vi "HTML Report Text Tag Attribute.vi"(0 "filter value (T)":bool=TRUE, 4 "default value (\"\")":string, 5 "value":string, 6 "label":string, 7 "tag attributes in":string) -> (3 "tag attributes out":string)   [LabVIEW 2020, in "NI_ReportGenerationCore.lvlib"]
doc: "For a value not equal to the default value, constructs the appropriate attribute."
uses:
  <vilib>/Utility/NIReport.llb/NI_ReportGenerationCore.lvlib
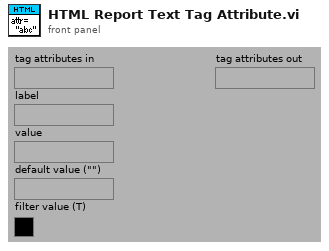
[diagram p1: front panel]
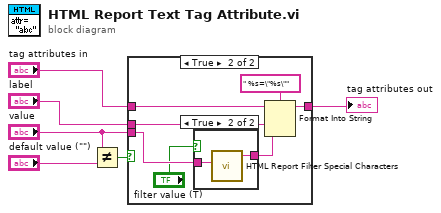
[diagram p0: block diagram]
diagram:
  n1 = Not Equal?(x="value", y="default value (\"\")") -> (x != y?=w3:bool)
  n2 = case shown="True" w3 {
    tunnel: [w7 w14] -> w5
    tunnel: "tag attributes in" -> [w7 w13]
    tunnel: "value" -> [_ w9]
    tunnel: "label" -> [_ w11]
    frame False {
    }
    frame True {
      n3 = case shown="True" "filter value (T)" {
        tunnel: w9 -> [w15 w17]
        tunnel: [w15 w16] -> w10
        frame False {
        }
        frame True {
          n4 = call <vilib>:"HTML Report Filter Special Characters.vi"("character string"=w17) -> ("HTML out"=w16:string)  [unwired: 2 in, 8 out]
        }
      }
      n5 = Format Into String(format string=" %s=\"%s\"", initial string=w13, w11, w10) -> (resulting string=w14:string)  [unwired: 1 in, 1 out]
    }
  }
  "tag attributes out" <- w5
